vi "vi_tree.vi"   [LabVIEW 2014, in "nanomsg.lvlib"]
uses:
  nanomsg.lvlib
  poll_event_data.ctl
  nanomsg_context.lvclass
  nanomsg_socket.lvclass
  nanomsg_getsocketopt_int.vi
  nanomsg_poll_scalar.vi
panel:
  # "See back-panel for VI tree"
types:
  T1 = typedef "nanomsg.lvlib/poll_event_data.ctl" = cluster{"identity":string, "data":string[]}
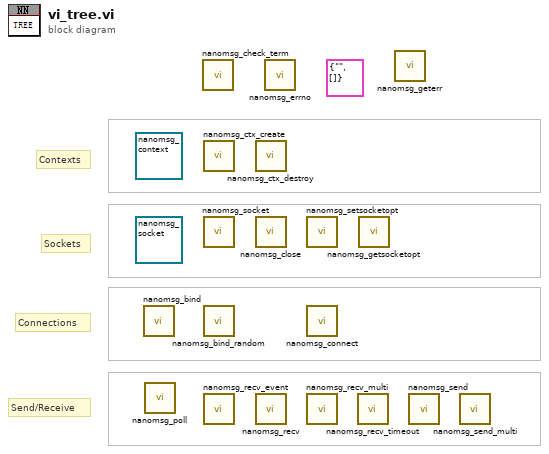
[diagram p0: block diagram]
diagram:
  (unwired) refnum<class "nanomsg_socket.lvclass"> refnum ("zeromq.lvlib:ZeroMQ Socket")
  (unwired) refnum<class "nanomsg_context.lvclass"> refnum ("zeromq.lvlib:ZeroMQ Context")
  (unwired) T1 {"identity"="", "data"=[]} ("poll data")
  # "Send/Receive"
  # "Connections"
  # "Sockets"
  # "Contexts"
  n1 = call "nanomsg_bind.vi"() -> ()  [unwired: 4 in, 2 out]
  n2 = call-poly "nanomsg_poll.vi"() -> ()  [unwired: 4 in, 4 out]
  n3 = call "nanomsg_check_term.vi"() -> ()  [unwired: 2 in, 2 out]
  n4 = call "nanomsg_ctx_create.vi"() -> ()  [unwired: 4 in, 2 out]
  n5 = call "nanomsg_socket.vi"() -> ()  [unwired: 5 in, 3 out]
  n6 = call "nanomsg_bind_random.vi"() -> ()  [unwired: 4 in, 4 out]
  n7 = call "nanomsg_recv_event.vi"() -> ()  [unwired: 7 in, 3 out]
  n8 = call "nanomsg_ctx_destroy.vi"() -> ()  [unwired: 5 in, 1 out]
  n9 = call "nanomsg_close.vi"() -> ()  [unwired: 5 in, 1 out]
  n10 = call "nanomsg_recv.vi"() -> ()  [unwired: 5 in, 5 out]
  n11 = call "nanomsg_errno.vi"() -> ()  [unwired: 2 in, 2 out]
  n12 = call "nanomsg_setsocketopt.vi"() -> ()  [unwired: 5 in, 2 out]
  n13 = call "nanomsg_connect.vi"() -> ()  [unwired: 4 in, 2 out]
  n14 = call "nanomsg_recv_multi.vi"() -> ()  [unwired: 3 in, 3 out]
  n15 = call "nanomsg_recv_timeout.vi"() -> ()  [unwired: 4 in, 4 out]
  n16 = call-poly "nanomsg_getsocketopt.vi"() -> ()  [unwired: 4 in, 3 out]
  n17 = call "nanomsg_geterr.vi"() -> ()  [unwired: 1 in, 1 out]
  n18 = call "nanomsg_send.vi"() -> ()  [unwired: 4 in, 2 out]
  n19 = call "nanomsg_send_multi.vi"() -> ()  [unwired: 4 in, 2 out]
